vi "RP100SetSlew.vi"(2 "error in (no error)":errorcluster, 3 "Voltage":dbl, 4 "Source":enum16{"1", "2", "Both"}(ring), 5 "VISA resource name":refnum<visa-resource-name>) -> (0 "error out":errorcluster, 1 "VISA resource name out":refnum<visa-resource-name>)   [LabVIEW 2020]
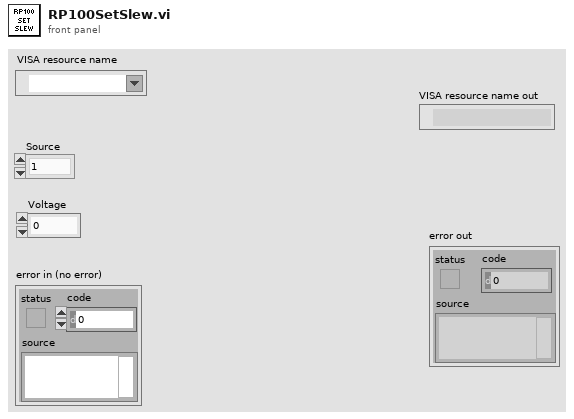
[diagram p1: front panel]
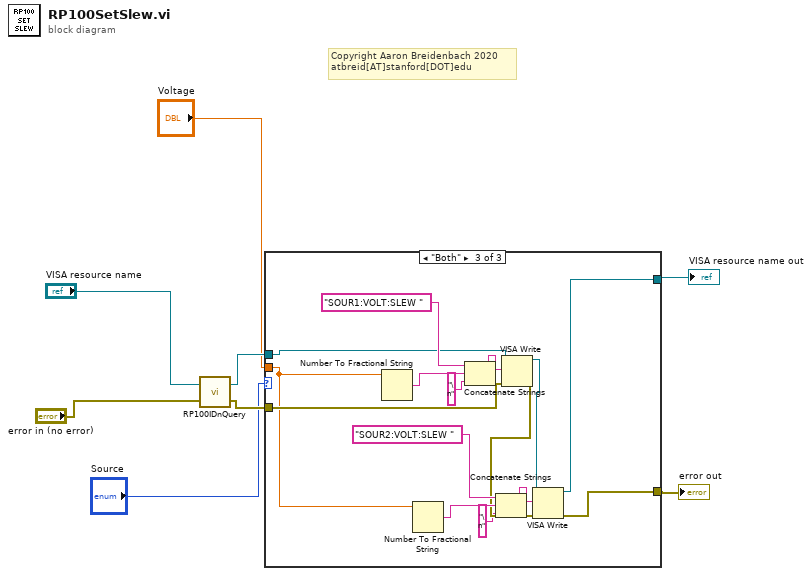
[diagram p0: block diagram]
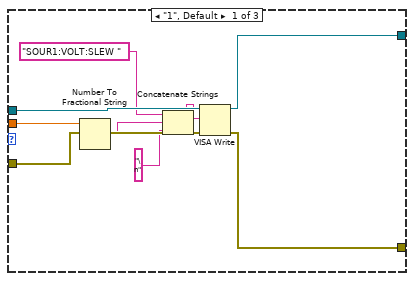
[diagram p2: hidden frame]
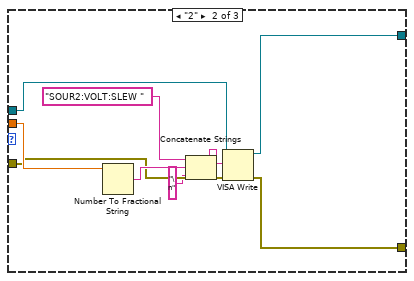
[diagram p3: hidden frame]
diagram:
  # "Copyright Aaron Breidenbach 2020\natbreid[AT]stanford[DOT]edu"
  n1 = call "RP100IDnQuery.vi"("error in (no error)"="error in (no error)", "VISA resource name"="VISA resource name") -> ("error out"=w8:errorcluster, "VISA resource name out"=w5:refnum<visa-resource-name>)
  n2 = case shown="\"Both\"" "Source" {
    tunnel: w5 -> [w17 w20 w35]
    tunnel: w8 -> [w16 w19 w32]
    tunnel: "Voltage" -> [w12 w21 w29]
    tunnel: [w9 w22 w33] -> w6
    tunnel: [w10 w23 w34] -> w7
    frame "1", Default {
      n3 = Number To Fractional String(number=w12) -> (F-format string=w14:string)  [unwired: 3 in]
      n4 = Concatenate Strings("SOUR1:VOLT:SLEW " ("write buffer"), w14, "\n" ("string")) -> (w15:string)
      n5 = VISA Write(VISA resource name=w17, write buffer=w15, error in (no error)=w16) -> (VISA resource name out=w10:refnum<visa-resource-name>, error out=w9:errorcluster)  [unwired: 1 out]
    }
    frame "2" {
      n6 = Number To Fractional String(number=w21) -> (F-format string=w25:string)  [unwired: 3 in]
      n7 = Concatenate Strings("SOUR2:VOLT:SLEW " ("write buffer"), w25, "\n" ("string")) -> (w26:string)
      n8 = VISA Write(VISA resource name=w20, write buffer=w26, error in (no error)=w19) -> (VISA resource name out=w23:refnum<visa-resource-name>, error out=w22:errorcluster)  [unwired: 1 out]
    }
    frame "Both" {
      n9 = Number To Fractional String(number=w29) -> (F-format string=w40:string)  [unwired: 3 in]
      n10 = Number To Fractional String(number=w29) -> (F-format string=w37:string)  [unwired: 3 in]
      n11 = Concatenate Strings("SOUR1:VOLT:SLEW " ("write buffer"), w40, "\n" ("string")) -> (w41:string)
      n12 = Concatenate Strings("SOUR2:VOLT:SLEW " ("write buffer"), w37, "\n" ("string")) -> (w38:string)
      n13 = VISA Write(VISA resource name=w35, write buffer=w41, error in (no error)=w32) -> (VISA resource name out=w31:refnum<visa-resource-name>, error out=w30:errorcluster)  [unwired: 1 out]
      n14 = VISA Write(VISA resource name=w31, write buffer=w38, error in (no error)=w30) -> (VISA resource name out=w34:refnum<visa-resource-name>, error out=w33:errorcluster)  [unwired: 1 out]
    }
  }
  "error out" <- w6
  "VISA resource name out" <- w7
